vi "TwGetStickSpectrumFromH5.vi"(0 "segmentIndex":i32, 1 "segmentEndIndex":i32, 2 "bufIndex":i32, 3 "bufEndIndex":i32, 4 "writeIndex":i32, 5 "writeEndIndex":i32, 6 "error in (no error)":errorcluster, 7 "spectrum in":sgl[](array[numeric]), 8 "filename":string, 9 "bufWriteLinked":u8, 11 "normalize":u8) -> (14 "error out":errorcluster, 19 "spectrum out":sgl[](array[numeric]))   [LabVIEW 2009]
uses:
  TwH5Dll.dll
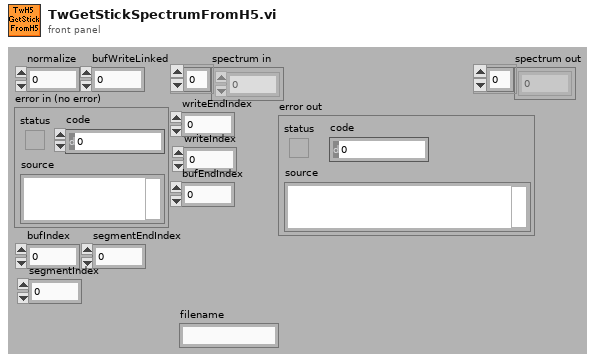
[diagram p1: front panel]
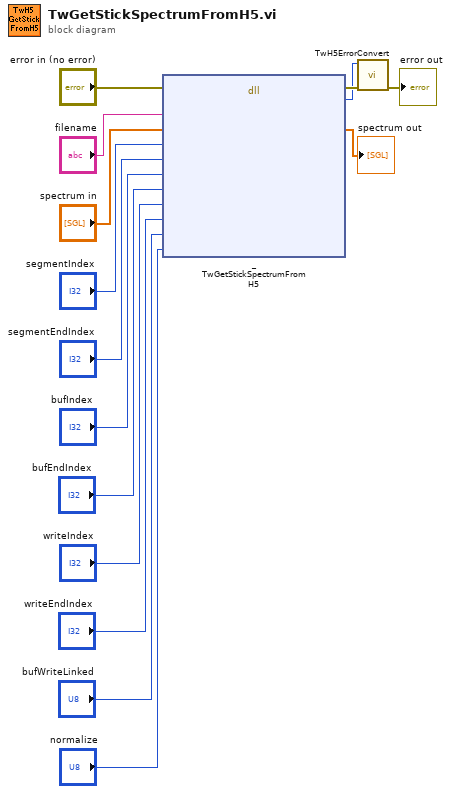
[diagram p0: block diagram]
diagram:
  n1 = dll-call lib="C:/src/85_TofDaq_current/DllWrappers/LabView/TwH5Dll/TwH5Dll.dll" fn="_TwGetStickSpectrumFromH5"(error in="error in (no error)", "filename"="filename", "spectrum"="spectrum in", "segmentIndex"="segmentIndex", "segmentEndIndex"="segmentEndIndex", "bufIndex"="bufIndex", "bufEndIndex"="bufEndIndex", "writeIndex"="writeIndex", "writeEndIndex"="writeEndIndex", "bufWriteLinked"="bufWriteLinked", "normalize"="normalize") -> (error out=w14:errorcluster, "TwRetVal"=w13:i32, "spectrum"=→"spectrum out":sgl[])  [unwired: 11 in, 1 out]
  n2 = call "TwH5ErrorConvert.vi"("error in (no error)"=w14, "error code"=w13) -> ("error out"=→"error out":errorcluster)  [unwired: 9 out]
